vi "Eval y=f(x) Optimal Step_core(VI).vi"(4 "sign":i32(ring) items=["y=f(x)", "y=-f(x)"], 5 "epsilon":dbl=0.05 min=1e-18 format="%.2f", 6 "data":variant, 7 "f(x)":T1, 8 "error in":i32, 9 "end":dbl=1.0 format="%.2f", 10 "start":dbl format="%.2f", 11 "number of points":u32=10) -> (0 "error out":i32, 1 "ticks":u32, 2 "Y Values":dbl[](array[numeric]) format="%.2f", 3 "X Values":dbl[](array[numeric]) format="%.2f")   [LabVIEW 2010, in "NI_Gmath.lvlib"]
uses:
  NI_Gmath.lvlib
  functionRefnum.ctl
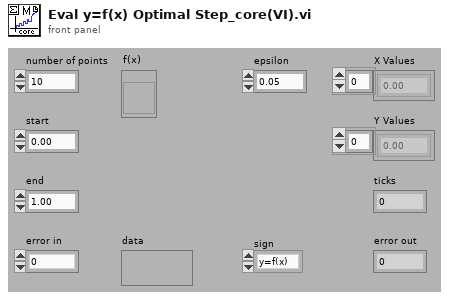
[diagram p1: front panel]
types:
  T1 = typedef "NI_Gmath.lvlib/functionRefnum.ctl" = refnum<vi>
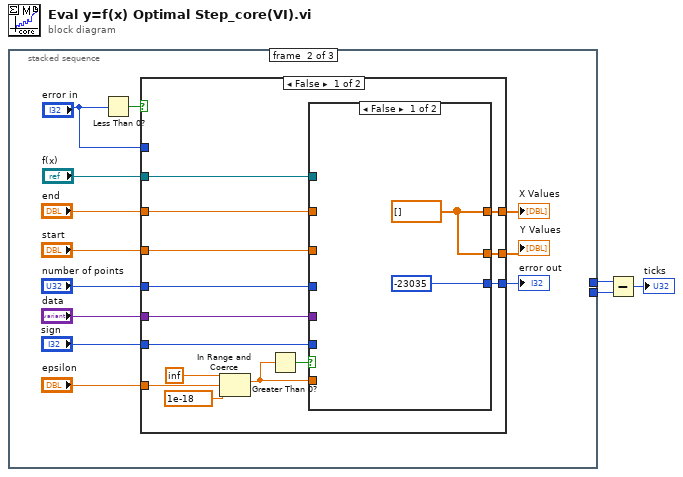
[diagram p0: block diagram]
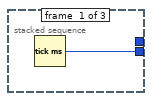
[diagram p2: hidden frame]
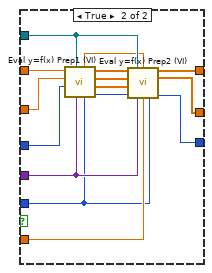
[diagram p3: hidden frame]
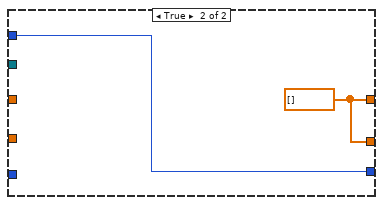
[diagram p4: hidden frame]
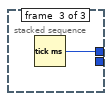
[diagram p5: hidden frame]
diagram:
  n1 = stacked-sequence {
    tunnel: [w4 _ _] -> w2
    tunnel: [_ _ w52] -> w1
    frame #0 {
      n2 = Tick Count (ms)() -> (millisecond timer value=w4:u32)
    }
    frame #1 {
      n3 = Less Than 0?(x="error in") -> (x < 0?=w13:bool)
      n4 = case shown="False" w13 {
        tunnel: [w30 w51] -> w16
        tunnel: [w25 w51] -> w15
        tunnel: [w24 w50] -> w14
        tunnel: "error in" -> [_ w50]
        tunnel: "f(x)" -> [w23 _]
        tunnel: "epsilon" -> [w22 _]
        tunnel: "data" -> [w21 _]
        tunnel: "sign" -> [w20 _]
        tunnel: "end" -> [w19 _]
        tunnel: "start" -> [w18 _]
        tunnel: "number of points" -> [w17 _]
        frame False {
          n5 = In Range and Coerce(upper limit=inf, x=w22, lower limit=1e-18) -> (coerced(x)=w26:dbl)  [unwired: 1 out]
          n6 = Greater Than 0?(x=w26) -> (x > 0?=w27:bool)
          n7 = case shown="False" w27 {
            tunnel: [w32 w46] -> w30
            tunnel: w26 -> [_ w45]
            tunnel: w21 -> [_ w44]
            tunnel: w23 -> [_ w43]
            tunnel: [w32 w42] -> w25
            tunnel: [-23035 w39] -> w24
            tunnel: w20 -> [_ w38]
            tunnel: w19 -> [_ w37]
            tunnel: w18 -> [_ w36]
            tunnel: w17 -> [_ w35]
            frame False {
              w32 = dbl[] [] ("X Values")
              (unwired) -23035
              (unwired) 0
              n8 = Initialize Array(0.0, 0) -> ()  [unwired: 1 out]
            }
            frame True {
              n9 = call "Eval y=f(x) Prep1 (VI).vi"("sign"=w38, "data"=w44, "f(x)"=w43, "number of points"=w35, "start"=w36, "end"=w37) -> ("error out"=w40:i32, "points II"=w47:dbl[], "points I"=w48:dbl[], "points"=w49:dbl[], "random summand"=w41:dbl)  [unwired: 1 in]
              n10 = call "Eval y=f(x) Prep2 (VI).vi"("points in"=w49, "f(x)"=w43, "random summand"=w41, "points I in"=w48, "points II in"=w47, "error in"=w40, "data"=w44, "epsilon"=w45, "sign"=w38) -> ("points out"=w42:dbl[], "points I out"=w46:dbl[], "error out"=w39:i32)  [unwired: 1 in, 3 out]
            }
          }
        }
        frame True {
          w51 = dbl[] [] ("points out")
        }
      }
      "X Values" <- w15
      "Y Values" <- w16
      "error out" <- w14
    }
    frame #2 {
      n11 = Tick Count (ms)() -> (millisecond timer value=w52:u32)
    }
  }
  n12 = Subtract(x=w1, y=w2) -> (x-y=→"ticks":u32)
